vi "CheckDPIDConfigurationforErrors.vi"(6 "Existing PIDs":T1[](array[typedef]) {"Signals"."Byte Order" items=["Little Endian", "Big Endian"]; "Signals"."Data Type" items=["Signed", "Unsigned", "IEEE Float"]}, 8 "error in (no error)":errorcluster, 9 "Existing DPIDs":u8[](array[numeric]), 10 "DPID ID":refnum<vi>, 11 "PIDs":refnum<vi>) -> (0 "error out":errorcluster, 2 "Reason":string, 3 "Error?":bool)   [LabVIEW 2015, in "Diagnostics Addon System Explorer.lvlib"]
uses:
  Diagnostics Addon System Explorer.lvlib
  Shared/Types/Frame Parameters.ctl
  Shared/Types/Signal Parameters.ctl
  Shared/Diagnostics Addon Shared.lvlib
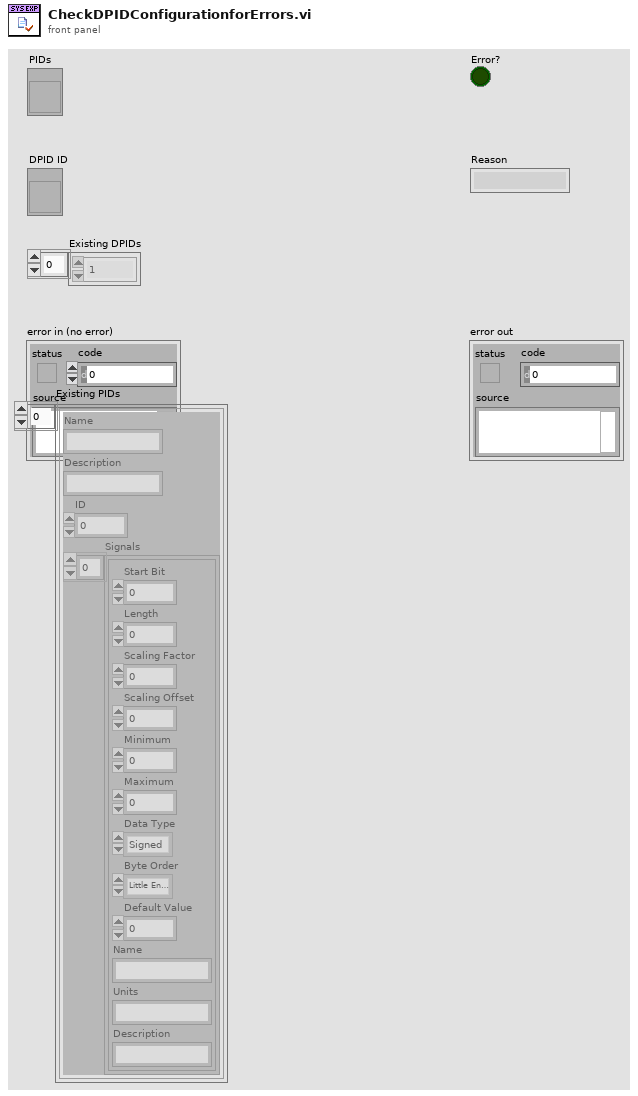
[diagram p1: front panel]
types:
  T1 = typedef "Diagnostics Addon Shared.lvlib/Frame Parameters.ctl" = cluster{"Name":string, "Description":string, "ID":u16, "Signals":T2[]}
  T2 = typedef "Diagnostics Addon Shared.lvlib/Signal Parameters.ctl" = cluster{"Start Bit":u8, "Length":u8, "Scaling Factor":dbl, "Scaling Offset":dbl, "Minimum":dbl, "Maximum":dbl, "Data Type":u32, "Byte Order":u32, "Default Value":dbl, "Name":string, "Units":string, "Description":string}
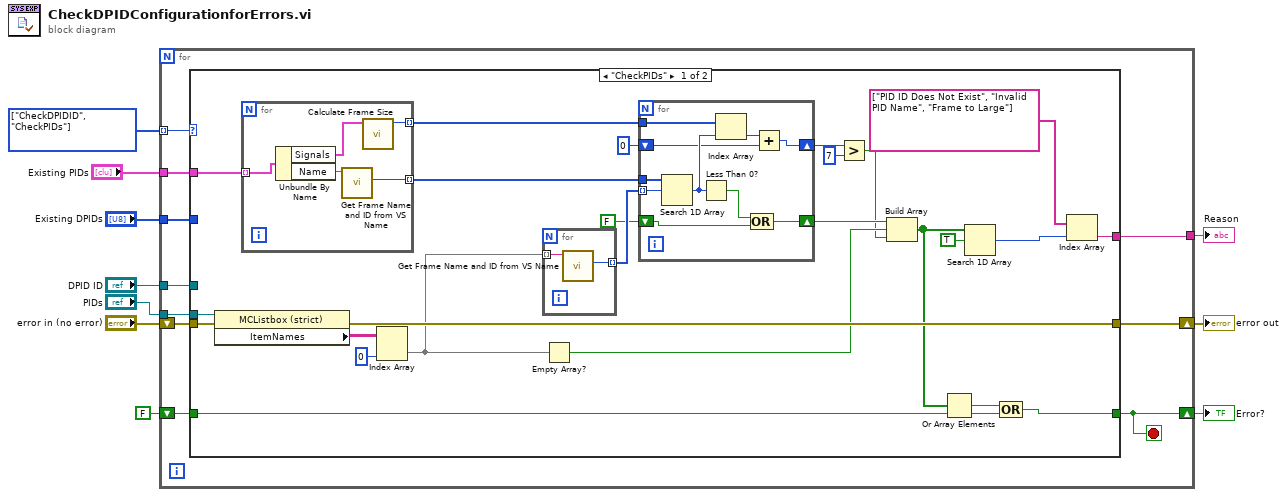
[diagram p0: block diagram]
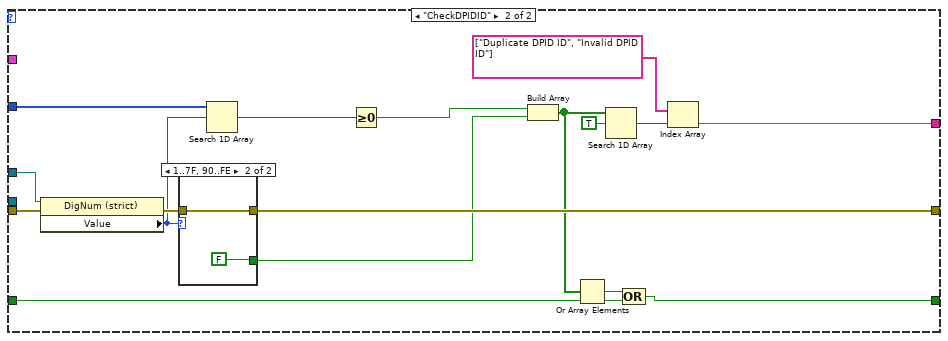
[diagram p2: hidden frame]
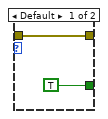
[diagram p3: hidden frame]
diagram:
  w10 = enum16{"CheckDPIDID", "CheckPIDs"}[] [enum."CheckDPIDID", enum."CheckPIDs"] items=["CheckDPIDID", "CheckPIDs"]
  n1 = for {
    tunnel: w10 -> [w20] mode=indexing
    shift-right: [w18] -> w7
    shift-left: "error in (no error)" -> [w19]
    tunnel: "PIDs" -> [w17]
    tunnel: "Existing DPIDs" -> [w16]
    shift-right: [w12] -> w3
    shift-left: FALSE -> [w15]
    tunnel: "DPID ID" -> [w14]
    tunnel: [w13] -> w2
    tunnel: "Existing PIDs" -> [w11]
    stop <- w12 stop-if-true
    n2 = case shown="\"CheckPIDs\"" w20 {
      tunnel: w19 -> [w43 w79]
      tunnel: [w42 w77] -> w18
      tunnel: w17 -> [w41 _]
      tunnel: w16 -> [_ w75]
      tunnel: [w37 w71] -> w12
      tunnel: w15 -> [w38 w72]
      tunnel: w14 -> [_ w78]
      tunnel: [w30 w63] -> w13
      tunnel: w11 -> [w26 _]
      frame "CheckPIDs" {
        n3 = property class="MCListbox (strict)"(reference=w41, error in=w43) -> (error out=w42:errorcluster, "ItemNames"=w45:string[][])  [unwired: 1 out]
        n4 = for {
          tunnel: [w50] -> w39 mode=indexing
          tunnel: w26 -> [w48] mode=indexing
          tunnel: [w47] -> w25 mode=indexing
          n5 = Unbundle By Name(w48) -> ("Signals"=w46:T2[], "Name"=w49:string)
          n6 = call "Get Frame Name and ID from VS Name.vi"("VS PID Name"=w49) -> ("ID"=w50:u16)  [unwired: 9 in, 1 out]
          n7 = call "Calculate Frame Size.vi"("Parameters"=w46) -> ("Bytes"=w47:u16)  [unwired: 10 in]
        }
        n8 = Index Array(array=w45, index (col)=0 ("disabled index (col)")) -> (element=w36:string[])  [unwired: 1 in]
        n9 = for {
          tunnel: w36 -> [w61] mode=indexing
          tunnel: [w62] -> w40 mode=indexing
          n10 = call "Get Frame Name and ID from VS Name.vi"("VS PID Name"=w61) -> ("ID"=w62:u16)  [unwired: 9 in, 1 out]
        }
        n11 = Empty Array?(array=w36) -> (empty?=w28:bool)
        n12 = for {
          tunnel: w39 -> [w60]
          tunnel: w40 -> [w59] mode=indexing
          shift-right: [w57] -> w32
          shift-left: FALSE -> [w56]
          tunnel: w25 -> [w55]
          shift-right: [w52] -> w23
          shift-left: u8 0 ("Frame Length") -> [w51]
          n13 = Search 1D Array(1D array=w60, element=w59) -> (index of element=w54:i32)  [unwired: 1 in]
          n14 = Less Than 0?(x=w54) -> (x < 0?=w58:bool)
          n15 = Index Array(array=w55, index=w54) -> (element=w53:u16)
          n16 = Compound Arithmetic op=OR(w58, w56) -> (w57:bool)
          n17 = Add(x=w53, y=w51) -> (x+y=w52:u16)
        }
        n18 = Greater?(x=w23, y=u8 7) -> (0:w21:bool)
        n19 = Build Array(w32, w28, w21) -> (w29:bool[])
        n20 = Or Array Elements(Boolean array=w29) -> (logical OR=w27:bool)
        n21 = Search 1D Array(1D array=w29, element=TRUE) -> (index of element=w34:i32)  [unwired: 1 in]
        n22 = Compound Arithmetic op=OR(w27, w38) -> (w37:bool)
        n23 = Index Array(array=string[] ["PID ID Does Not Exist", "Invalid PID Name", "Frame to Large"], index=w34) -> (element=w30:string)
      }
      frame "CheckDPIDID" {
        n24 = property class="DigNum (strict)"(reference=w78, error in=w79) -> (error out=w76:errorcluster, "Value"=w74:u8)  [unwired: 1 out]
        n25 = case shown="1..7F, 90..FE" w74 {
          tunnel: [w81 w83] -> w77
          tunnel: w76 -> [w81 w83]
          tunnel: [TRUE FALSE] -> w65
          frame Default {
          }
          frame 1..127, 144..254 {
          }
        }
        n26 = Search 1D Array(1D array=w75, element=w74) -> (index of element=w73:i32)  [unwired: 1 in]
        n27 = Greater Or Equal To 0?(x=w73) -> (x >= 0?=w66:bool)
        n28 = Build Array(w66, w65) -> (w67:bool[])
        n29 = Or Array Elements(Boolean array=w67) -> (logical OR=w64:bool)
        n30 = Search 1D Array(1D array=w67, element=TRUE) -> (index of element=w69:i32)  [unwired: 1 in]
        n31 = Compound Arithmetic op=OR(w64, w72) -> (w71:bool)
        n32 = Index Array(array=string[] ["Duplicate DPID ID", "Invalid DPID ID"], index=w69) -> (element=w63:string)
      }
    }
  }
  "error out" <- w7
  "Error?" <- w3
  "Reason" <- w2
